vi "asset.get.vi"(8 "error in (no error)":errorcluster, 11 "Run in":refnum<class "Run.lvclass">) -> (0 "error out":errorcluster, 2 "Asset":refnum<class "asset.lvclass">, 3 "Run out":refnum<class "Run.lvclass">)   [LabVIEW 2020, in "Run.lvclass"]
uses:
  Run.lvclass
  Run.lvclass/Run.ctl
  de85e14f-50dd-4ec2-a9b0-0cc4386a757e.vi
  de85e14f-50dd-4ec2-a9b0-0cc4386a757e.vi/32c3acc2-0975-485a-8283-62feb0f3dc4f.vi
  run_properties.get.vi
  <vilib>/JDP Science/JSONtext/JSON type.vi
  <vilib>/JDP Science/JSONtext/JSON text to Variant.vi
  <vilib>/JDP Science/JSONtext/LVClass Serializer/JSONtext LVClass Serializer.lvclass
  Nominal Client/Nominal Client.lvclass
  asset/asset.lvclass
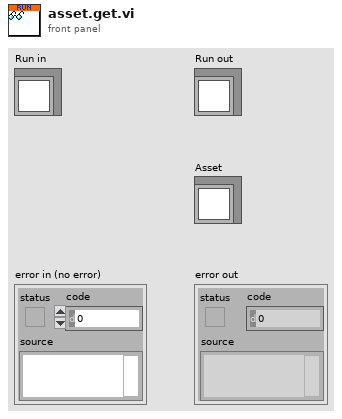
[diagram p1: front panel]
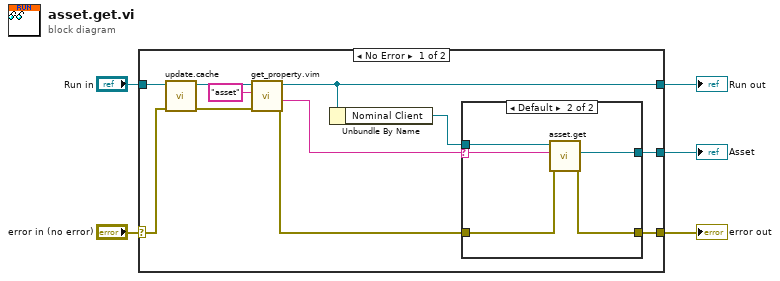
[diagram p0: block diagram]
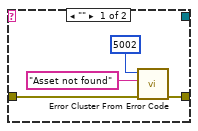
[diagram p2: hidden frame]
diagram:
  n1 = case shown="No Error" "error in (no error)" {
    selector: "error in (no error)" -> [w16 w26]
    tunnel: [w7 w26] -> w4
    tunnel: [w9 w27] -> w2
    tunnel: "Run in" -> [w15 w27]
    tunnel: [w6 _] -> w1
    frame No Error {
      n2 = call "update.cache.vi"("error in"=w16, "Run in"=w15) -> ("error out"=w12:errorcluster, "Run out"=w14:refnum<class "Run.lvclass">)  [unwired: 8 in]
      n3 = call "get_property.vim"("error in"=w12, "Property Name"="asset", "Run in"=w14) -> ("error out"=w8:errorcluster, "Value"=w11:string, "Run out"=w9:refnum<class "Run.lvclass">)  [unwired: 6 in]
      n4 = Unbundle By Name(w9) -> ("Nominal Client"=w10:refnum<class "Nominal Client.lvclass">)
      n5 = case shown="Default" w11 {
        selector: w11 -> [_ w25]
        tunnel: w10 -> [_ w24]
        tunnel: w8 -> [w19 w23]
        tunnel: [w20 w22] -> w7
        tunnel: [_ w21] -> w6
        frame "" {
          n6 = call <vilib>:"Error Cluster From Error Code.vi"("error in (no error)"=w19, "error message (\"\")"="Asset not found" ("error message (\"\")"), "error code (0)"=5002) -> ("error out"=w20:errorcluster)  [unwired: 6 in]
        }
        frame Default {
          n7 = call "asset.get.vi"("error in"=w23, "Asset RID"=w25, "Nominal Client in"=w24) -> ("error out"=w22:errorcluster, "Asset"=w21:refnum<class "asset.lvclass">)  [unwired: 6 in, 1 out]
        }
      }
    }
    frame Error {
    }
  }
  "error out" <- w4
  "Run out" <- w2
  "Asset" <- w1
